vi "Get Yaw.vi"() -> (0 "Angle":dbl)   [LabVIEW 2015]
uses:
  Robot Global Data.vi
  <vilib>/Rock Robotics/Network Tables/SD Write Number.vi
  navXLibraryv2.lvlibp
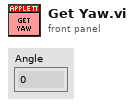
[diagram p1: front panel]
types:
  T1 = typedef "navXLibraryv2.lvlibp/Z900_navX_DeviceTypeDef.ctl" = cluster{"Interface":cluster{"Protocol":T2, "Update Rate (4Hz-60Hz)":u8, "navX Open TypeDef":variant}, "Notify Packet":refnum<notifier>, "Loop VI Refnum":refnum<vi>, "Ready to Close Occurrence Refnum":refnum<k4>}
  T2 = typedef "navXLibraryv2.lvlibp/Z900_navX_ProtocolTypeDef.ctl" = enum16{"SERIAL", "I2C", "SPI"}
  T3 = cluster{"Yaw":dbl, "Roll":dbl, "Pitch":dbl, "Heading":dbl, "Fused Heading":dbl}
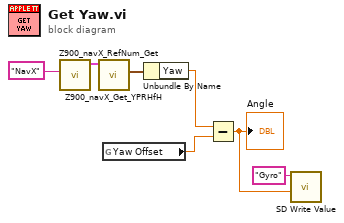
[diagram p0: block diagram]
diagram:
  n1 = call "Z900_navX_RefNum_Get.vi"("refnum name"="NavX") -> ("navX Device"=w2:T1)  [unwired: 9 in, 1 out]
  n2 = call "Z900_navX_Get_YPRHfH.vi"("navX Device"=w2) -> ("YRPHfH"=w1:T3)  [unwired: 7 in, 3 out]
  n3 = global read "Robot Global Data.vi" "Yaw Offset"() -> (w7:dbl)
  n4 = Unbundle By Name(w1) -> ("Yaw"=w6:dbl)
  n5 = Subtract(x=w6, y=w7) -> (x-y=w5:dbl)
  "Angle" <- w5
  n6 = call-poly <vilib>:"SD Write Value.vi"("Numeric"=w5, "Name"="Gyro") -> ()  [unwired: 8 in, 2 out]
